vi "get_single_acq.vi"(8 "error in (no error)":errorcluster, 11 "Stresing_dual_cam in":refnum<class "Stresing_dual_cam.lvclass">) -> (0 "error out":errorcluster, 1 "wavelengths":dbl[](array[numeric]), 2 "intensity":dbl[][](array[numeric]) format="%.2f", 3 "Stresing_dual_cam out":refnum<class "Stresing_dual_cam.lvclass">, 4 "trig channel 2":bool[](array[boolean]), 6 "trig channel 1":bool[](array[boolean]))   [LabVIEW 2019, in "Stresing_dual_cam.lvclass"]
uses:
  Stresing_dual_cam.lvclass
  _cameraBase/_cameraBase.lvclass
panel:
  out "Numeric":i32
  out "data_raw_sig":u16[][](array[numeric])
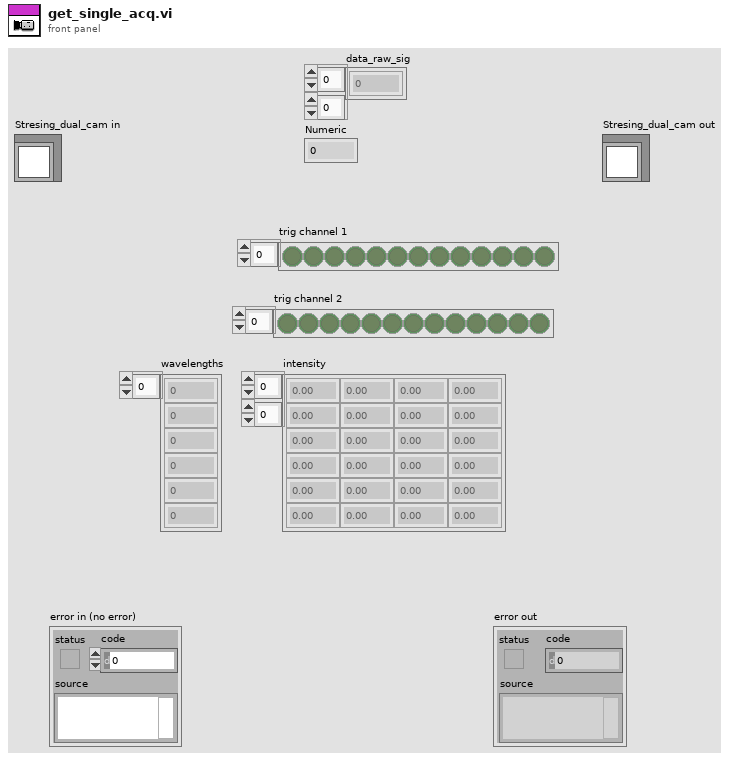
[diagram p1: front panel]
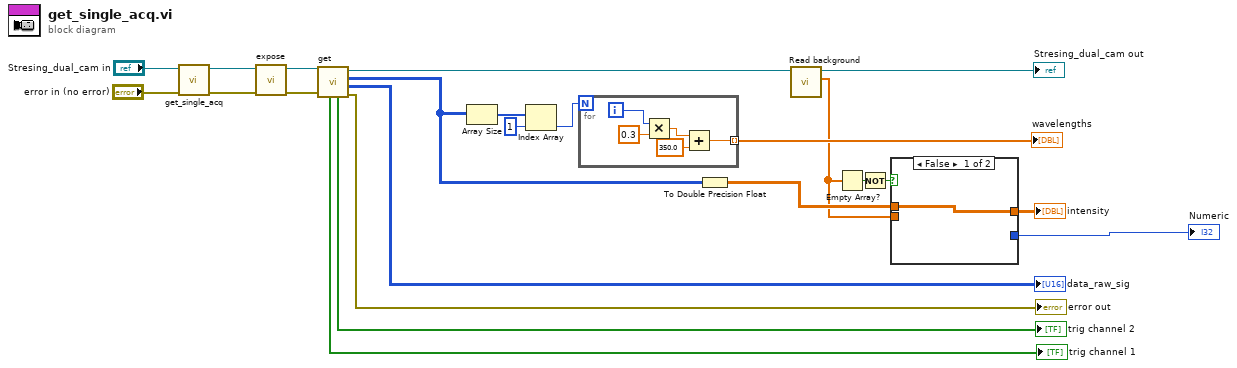
[diagram p0: block diagram]
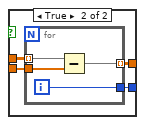
[diagram p2: hidden frame]
diagram:
  n1 = call-parent "get_single_acq.vi"("error in (no error)"="error in (no error)", "_cameraBase in"="Stresing_dual_cam in") -> ("error out"=w21:errorcluster, "_cameraBase out"=w20:refnum<class "Stresing_dual_cam.lvclass">)  [unwired: 4 in, 4 out]
  n2 = call-dynamic "expose.vi"("error in (no error)"=w21, "Stresing_dual_cam in"=w20) -> ("error out"=w18:errorcluster, "Stresing_dual_cam out"=w19:refnum<class "Stresing_dual_cam.lvclass">)  [unwired: 8 in]
  n3 = call-dynamic "get.vi"("error in (no error)"=w18, "Stresing_dual_cam in"=w19) -> ("error out"=→"error out":errorcluster, "data_raw_sig"=→"data_raw_sig":u16[][], "data_raw_ref"=w13:u16[][], "Stresing_dual_cam out"=w8:refnum<class "Stresing_dual_cam.lvclass">, "chop_sig"=→"trig channel 2":bool[], "chop_ref"=→"trig channel 1":bool[])  [unwired: 4 in]
  n4 = Array Size(array=w13) -> (size(s)=w12:i32[])
  n5 = Index Array(array=w12, index=1) -> (element=w10:i32)
  n6 = for {
    N: w10 -> [_]
    tunnel: [w24] -> w9 mode=indexing
    i -> [w28]
    n7 = Multiply(x=w28, y=0.3) -> (x*y=w26:dbl)
    n8 = Add(x=w26, y=350.0) -> (x+y=w24:dbl)
  }
  "wavelengths" <- w9
  n9 = To Double Precision Float(number=w13) -> (double precision float=w6:dbl[][])
  n10 = call-dynamic "Read background.vi"("_cameraBase in"=w8) -> ("background"=w3:dbl[], "_cameraBase out"=→"Stresing_dual_cam out":refnum<class "Stresing_dual_cam.lvclass">)  [unwired: 8 in, 1 out]
  n11 = Empty Array?(array=w3) -> (empty?=w1:bool)
  n12 = Not(x=w1) -> (.not. x?=w2:bool)
  n13 = case shown="False" w2 {
    tunnel: w6 -> [w29 w33]
    tunnel: w3 -> [_ w32]
    tunnel: [w29 w31] -> w5
    tunnel: [_ w30] -> w4
    frame False {
    }
    frame True {
      n14 = for {
        tunnel: w33 -> [w37] mode=indexing
        tunnel: w32 -> [w36]
        tunnel: [w35] -> w31 mode=indexing
        tunnel: [w34] -> w30
        i -> [w34]
        n15 = Subtract(x=w37, y=w36) -> (x-y=w35:dbl[])
      }
    }
  }
  "intensity" <- w5
  "Numeric" <- w4
